vi "Read Upload ID.vi"(8 "error in (no error)":errorcluster, 11 "Multipart Upload in":refnum<class "Multipart Upload.lvclass">) -> (0 "error out":errorcluster, 2 "Upload ID":string, 3 "Multipart Upload out":refnum<class "Multipart Upload.lvclass">)   [LabVIEW 2015, in "NI_AWS_S3.lvlib" / "Multipart Upload.lvclass"]
uses:
  Multipart Upload.lvclass
  Multipart Upload.lvclass/Multipart Upload.ctl
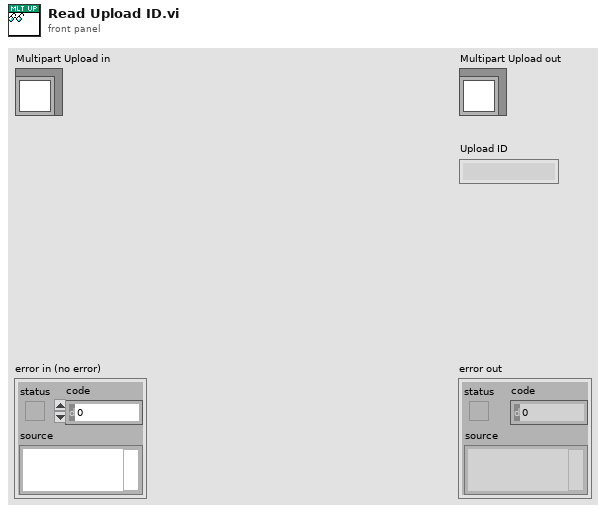
[diagram p1: front panel]
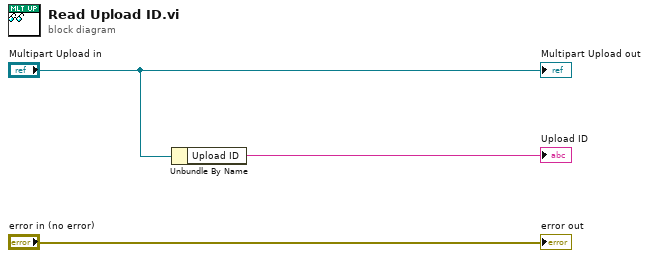
[diagram p0: block diagram]
diagram:
  n1 = Unbundle By Name("Multipart Upload in") -> ("Upload ID"=→"Upload ID":string)
  "error out" <- "error in (no error)"
  "Multipart Upload out" <- "Multipart Upload in"
